vi "lvEtherbone.test_snoop.vi"() -> ()   [LabVIEW 2009, in "lvEtherbone.lvlib"]
doc: "This example performs a multiple read/write _one_ Etherbone device and does this multiple times. This can be used to determine the average time of transactions."
uses:
  lvEtherbone.lvlib
  lvEtherbone.eb_mode_t.ctl
  lvEtherbone.lveb_status_t.ctl
panel:
  out "timePerIteration":dbl
  in  "nOfIterations":i32=1
  out "timed out?":bool
  out "eb_status":T1
  in  "dataW":u64[](array[numeric])=[291] format="%.0x"
  in  "modeW":T2 items=["EB_UNDEFINED"=-1, "EB_FIFO"=0, "EB_LINEAR"=1]
  in  "addressW":u64=32768 format="%.0x"
  in  "nR":i32
  in  "modeR":T2 items=["EB_UNDEFINED"=-1, "EB_FIFO"=0, "EB_LINEAR"=1]
  out "dataR":u64[](array[numeric]) format="%.0x"
  in  "addressR":u64=32776 format="%.0x"
  in  "timeout [ms]":i32=1000
  in  "ip_port":string="111.222.333.444:5555"
  out "error out":errorcluster
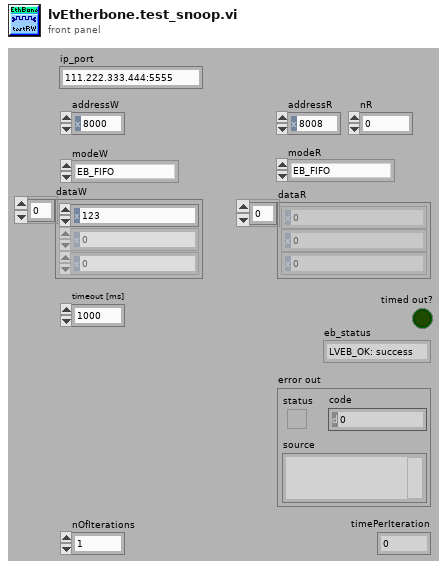
[diagram p1: front panel]
types:
  T1 = typedef "lvEtherbone.lvlib/lvEtherbone.lveb_status_t.ctl" = enum32{"LVEB_OK: success", "LVEB_UNKNOWN: unknown error", "LVEB_OS: operating system forbids access", "LVEB_PORT: port in use or unavailable", "LVEB_ID: ID invalid or out of resources", "LVEB_SOCKET: socket invalid or unavailable", "LVEB_EB: remote address is not Etherbone conformant", "LVEB_IP: bad format or network address", "LVEB_PORTWIDTH: port width error", "LVEB_DEVICEBUSY: Etherbone device still busy", "LVEB_DEVICEFAIL: operation on Wishbone device failed", "LVEB_DEVICEEXIST: Etherbone device already exists, overlaps, or does not exist", "LVEB_TIMEDOUT: a timeout occurred", "LVEB_OVERFLOW: payload of Etherbone exceeded", "LVEB_ADDRESS: bad address", "LVEB_ADDRESSWIDTH: address width error"}
  T2 = typedef "lvEtherbone.lvlib/lvEtherbone.eb_mode_t.ctl" = i32
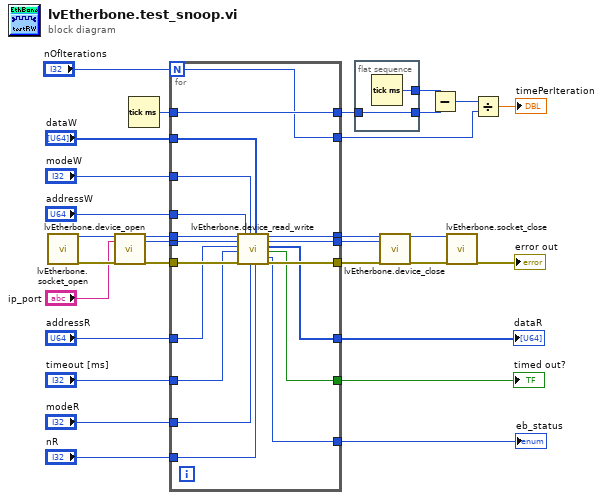
[diagram p0: block diagram]
diagram:
  n1 = call "lvEtherbone.socket_open.vi"() -> ("eb_socket_ID"=w2:i32, "error out"=w29:errorcluster)  [unwired: 17 in, 1 out]
  n2 = call "lvEtherbone.device_open.vi"("eb_socket_ID"=w2, "ip_port"="ip_port", "error in (no error)"=w29) -> ("eb_socket_ID out"=w23:i32, "eb_device_ID"=w1:i32, "error out"=w28:errorcluster)  [unwired: 12 in, 2 out]
  n3 = Tick Count (ms)() -> (millisecond timer value=w9:u32)
  n4 = for {
    N: "nOfIterations" -> [w31]
    tunnel: w28 -> [w48]
    tunnel: [w47] -> w27
    tunnel: w1 -> [w46]
    tunnel: "timeout [ms]" -> [w45]
    tunnel: w23 -> [w44]
    tunnel: [w43] -> w22
    tunnel: [w42] -> w20
    tunnel: "addressR" -> [w41]
    tunnel: [w40] -> w18
    tunnel: "modeR" -> [w39]
    tunnel: "nR" -> [w38]
    tunnel: "addressW" -> [w37]
    tunnel: "modeW" -> [w36]
    tunnel: "dataW" -> [w35]
    tunnel: [w34] -> w12
    tunnel: [w33] -> w11
    tunnel: w9 -> [w32]
    tunnel: [w32] -> w8
    tunnel: [w31] -> w4
    n5 = call "lvEtherbone.device_read_write.vi"("eb_socket_ID"=w44, "eb_device_ID"=w46, "addressR"=w41, "timeout [ms]"=w45, "error in (no error)"=w48, "addressW"=w37, "modeW"=w36, "modeR"=w39, "dataW"=w35, "nR"=w38) -> ("eb_status"=w34:T1, "eb_socket_ID out"=w43:i32, "eb_device_ID out"=w42:i32, "dataR"=w40:u64[], "timed out?"=w33:bool, "error out"=w47:errorcluster)  [unwired: 4 in]
  }
  "dataR" <- w18
  "eb_status" <- w12
  "timed out?" <- w11
  n6 = flat-sequence {
    tunnel: w8 -> [w50]
    tunnel: [w50] -> w7
    tunnel: [w49] -> w6
    frame #0 {
      n7 = Tick Count (ms)() -> (millisecond timer value=w49:u32)
    }
  }
  n8 = call "lvEtherbone.device_close.vi"("eb_socket_ID"=w22, "eb_device_ID"=w20, "error in (no error)"=w27) -> ("eb_socket_ID out"=w21:i32, "error out"=w26:errorcluster)  [unwired: 14 in, 1 out]
  n9 = Subtract(x=w6, y=w7) -> (x-y=w5:u32)
  n10 = call "lvEtherbone.socket_close.vi"("eb_socket_ID"=w21, "error in (no error)"=w26) -> ("error out"=→"error out":errorcluster)  [unwired: 16 in, 1 out]
  n11 = Divide(x=w5, y=w4) -> (x/y=→"timePerIteration":dbl)
